vi "Build All TWM Versions.vi"() -> ()   [LabVIEW 2020]
doc: "This VI will automatically build selected versions (different driver sets, etc.)."
uses:
  <vilib>/AppBuilder/AB_API_Simple/Build Specification Version.ctl
  Build Setup.ctl
  1a084e9b-14bd-426b-b511-56d3df6ad0ad.vi
  <vilib>/Utility/error.llb/Error Cluster From Error Code.vi
  <vilib>/AppBuilder/AB_API_Simple/Get Build Specification Version (path).vi
  <vilib>/AppBuilder/AB_API_Simple/Set Build Specification Version (path).vi
  <vilib>/ErrorRing/Error Ring.xnode
  <vilib>/Comparison/Equal/Equal Functor/Equal Functor.lvclass
  <vilib>/AppBuilder/AB_API_Simple/NI_App_Builder_API.lvlib
panel:
  in  "btn exit":bool
  in  "Build Specification Version (editable)":T1
  in  "build regexp filter":string="TWM -" caption="Build Specification regexp Filter (e.g.: \"TWM-\" or \".*\" for no filtering)"
  out "Status":string
  in  "btn all":bool
  in  "builds":i32[](listbox) caption="Available build variants (different configuration sets, select some for build):"
  in  "Target Name":string="My Computer" caption="Target Name (typically \"My Computer\")"
  in  "full build name":string="TWM - full" caption="Build Specification Name (the fully equiped version)"
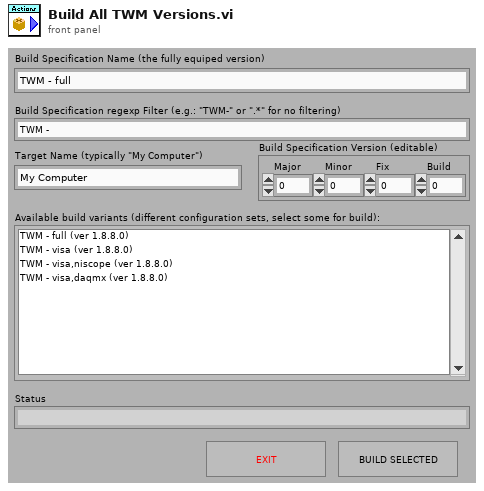
[diagram p1: front panel]
types:
  T1 = typedef "NI_App_Builder_API.lvlib/Build Specification Version.ctl" = cluster{"Major":u16, "Minor":u16, "Fix":u16, "Build":u16}
  T2 = typedef "Build Setup.ctl" = cluster{"project path":path, "build spec name":string, "target name":string}
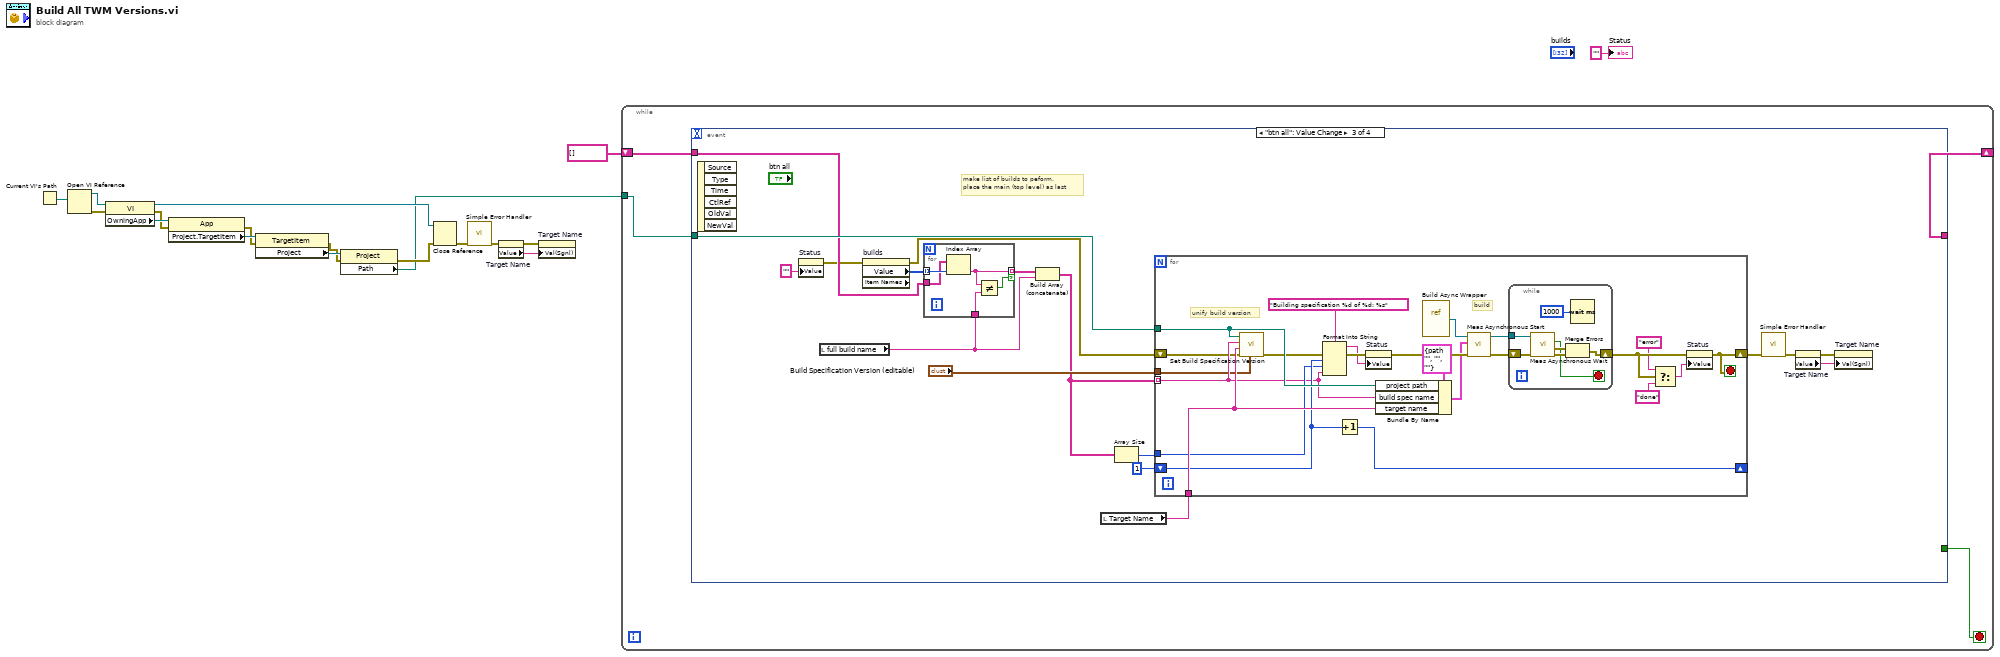
[diagram p0: block diagram]
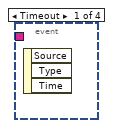
[diagram p2: hidden frame]
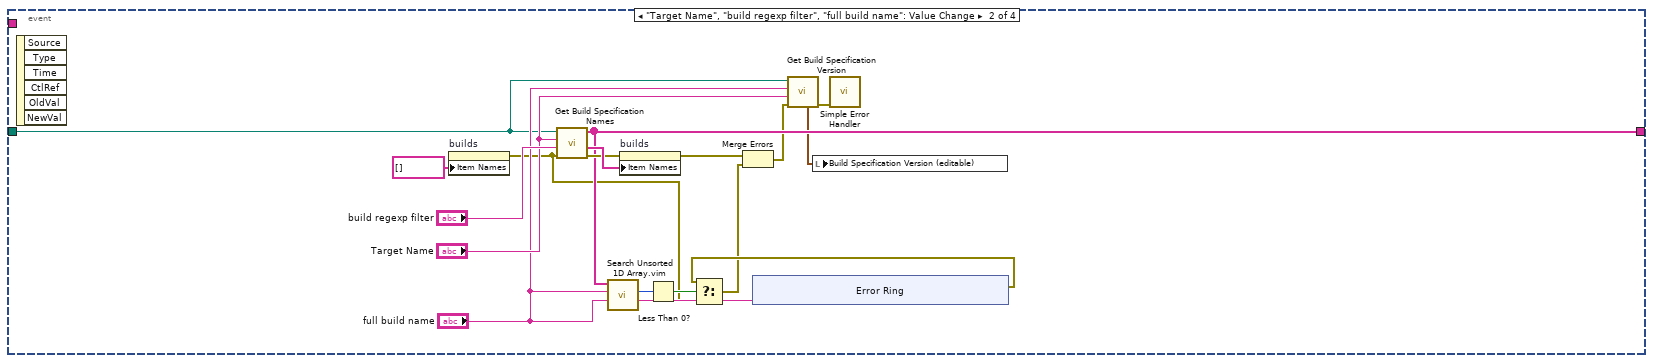
[diagram p3: hidden frame]
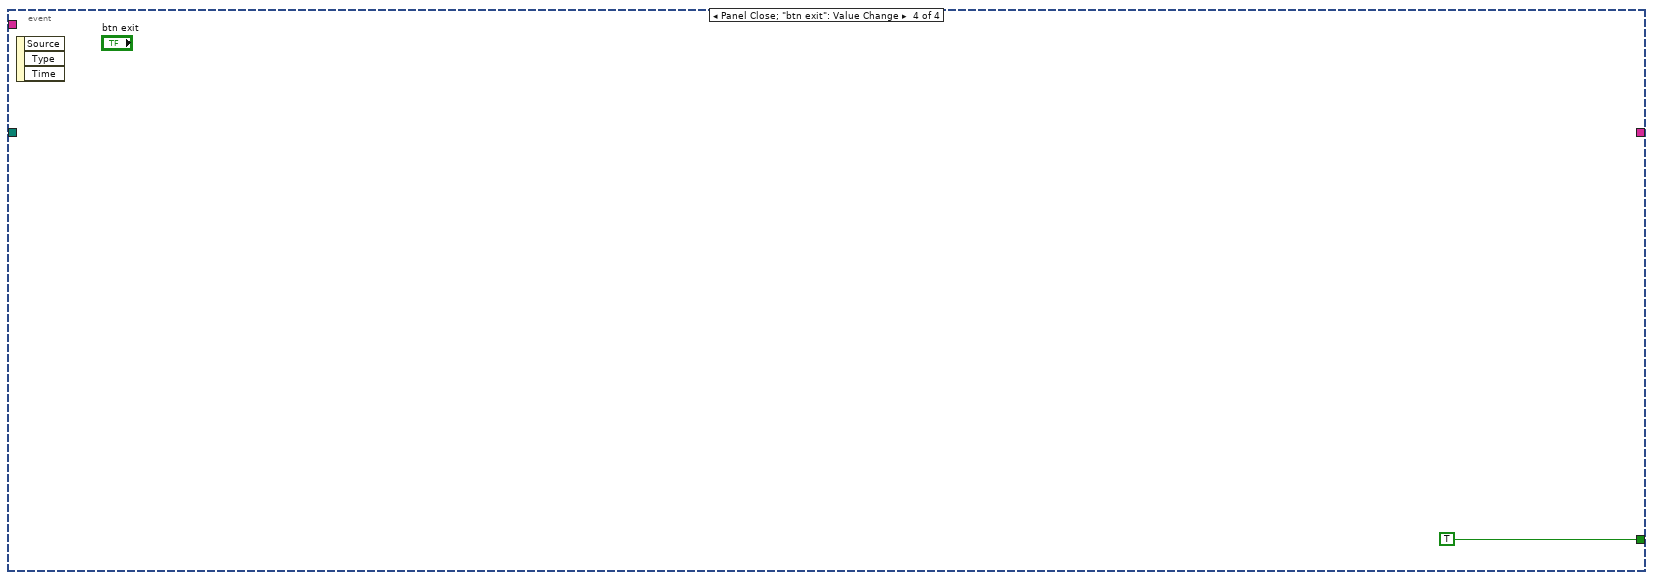
[diagram p4: hidden frame]
diagram:
  n1 = Current VI's Path() -> (path=w17:path)
  n2 = Open VI Reference(vi path=w17) -> (vi reference=w15:refnum<vi>, error out=w16:errorcluster)  [unwired: 5 in]
  n3 = property class="VI"(reference=w15, error in=w16) -> (reference out=w10:refnum<vi>, error out=w13:errorcluster, "OwningApp"=w14:refnum<vi>)
  n4 = property class="App"(reference=w14, error in=w13) -> (error out=w11:errorcluster, "Project.TargetItem"=w12:refnum<vi>)  [unwired: 1 out]
  n5 = property class="TargetItem"(reference=w12, error in=w11) -> (error out=w8:errorcluster, "Project"=w9:refnum<vi>)  [unwired: 1 out]
  n6 = property class="Project"(reference=w9, error in=w8) -> (error out=w7:errorcluster, "Path"=w6:path)  [unwired: 1 out]
  n7 = Close Reference(reference=w10, error in (no error)=w7) -> (error out=w5:errorcluster)
  n8 = call <vilib>:"Simple Error Handler.vi"("error in (no error)"=w5) -> ("error out"=w3:errorcluster)  [unwired: 4 in, 4 out]
  n9 = property on="Target Name" class="Str"(error in=w3) -> (error out=w1:errorcluster, "Value"=w2:string)  [unwired: 1 in, 1 out]
  n10 = property on="Target Name" class="Str"(error in=w1, "Val(Sgnl)"=w2) -> ()  [unwired: 1 in, 2 out]
  n11 = while {
    tunnel: w6 -> [w22]
    shift-right: [w21] -> _
    shift-left: string[] [] ("Build specification names") -> [w20]
    stop <- w19 stop-if-true
    n12 = event shown="[2] \"btn all\": Value Change" {
      selector: _ -> [_ _ _ _]
      dyn-events: _ -> [_ _ _ _]
      timeout: _ -> [_ _ _ _]
      tunnel: [_ w35 _ _] -> w21
      tunnel: w22 -> [_ w26 w54 _]
      tunnel: w20 -> [_ _ w52 _]
      tunnel: [_ _ _ TRUE] -> w19
      event Timeout {
        n13 = event-data() -> ()  [unwired: 1 in, 3 out]
      }
      event "Target Name", "build regexp filter", "full build name": Value Change {
        n14 = event-data() -> ()  [unwired: 1 in, 6 out]
        n15 = property on="builds" class="LstBox (strict)"("Item Names"=string[] []) -> (error out=w27:errorcluster)  [unwired: 2 in, 1 out]
        n16 = call "Get Build Specification Names.vi"("error in (no error)"=w27, "Build specification regexp filter (.*)"="build regexp filter", "Target Name"="Target Name", "Project Path"=w26) -> ("error out"=w38:errorcluster, "Build specification names with version string"=w39:string[], "Build specification names"=w35:string[])  [unwired: 3 in, 2 out]
        n17 = call "Search Unsorted 1D Array.vim"("element"="full build name", "unsorted 1D array"=w35) -> ("index of element"=w32:i32)  [unwired: 9 in]
        n18 = property on="builds" class="LstBox (strict)"(error in=w38, "Item Names"=w39) -> (error out=w29:errorcluster)  [unwired: 1 in, 1 out]
        n19 = Less Than 0?(x=w32) -> (x < 0?=w31:bool)
        n20 = xnode "Error Ring"("parameter 0"="full build name") -> ("error out"=w30:errorcluster)
        n21 = Select(t=w30, s=w31, f=w27) -> (s? t:f=w28:errorcluster)
        n22 = Merge Errors(w29, w28) -> (w25:errorcluster)
        n23 = call-poly <vilib>:"Get Build Specification Version.vi"("error in (no error)"=w25, "Name of target (My Computer)"="Target Name", "Name of build specification"="full build name", "Path to project"=w26) -> ("error out"=w24:errorcluster, "Build Specification Version"=w23:T1)  [unwired: 6 in]
        n24 = local write "Build Specification Version (editable)"(w23) -> ()
        n25 = call <vilib>:"Simple Error Handler.vi"("error in (no error)"=w24) -> ()  [unwired: 4 in, 5 out]
      }
      event "btn all": Value Change {
        # "make list of builds to peform,\nplace the main (top level) as last"
        n26 = event-data() -> ()  [unwired: 1 in, 6 out]
        n27 = property on="Status" class="Str"("Value"="" ("Status")) -> (error out=w48:errorcluster)  [unwired: 2 in, 1 out]
        n28 = local read "full build name"() -> (w62:string)
        n29 = property on="builds" class="LstBox (strict)" props=["Value", "Item Names"](error in=w48) -> (error out=w60:errorcluster, "Value"=w56:i32[])  [unwired: 1 in, 2 out]
        n30 = for {
          tunnel: w56 -> [w98] mode=indexing
          tunnel: w52 -> [w97]
          tunnel: w62 -> [w96]
          tunnel: [w95] -> w58 mode=indexing if=w94
          n31 = Index Array(array=w97, index=w98) -> (element=w95:string)
          n32 = Not Equal?(x=w95, y=w96) -> (x != y?=w94:bool)
        }
        n33 = Build Array (concatenate)(w58, w62) -> (w59:string[])
        n34 = local read "Target Name"() -> (w63:string)
        n35 = Array Size(array=w59) -> (size(s)=w57:i32)
        n36 = for {
          tunnel: w54 -> [w86]
          tunnel: w63 -> [w85]
          tunnel: w59 -> [w71] mode=indexing
          tunnel: w57 -> [w72]
          shift-right: [w84] -> _
          shift-left: 1 -> [w73]
          shift-right: [w68] -> w55
          shift-left: w60 -> [w69]
          tunnel: "Build Specification Version (editable)" -> [w70]
          stop <- w68 stop-if-true
          # "build"
          # "unify build version"
          n37 = call-poly <vilib>:"Set Build Specification Version.vi"("Build Specification Version"=w70, "error in (no error)"=w69, "Name of target (My Computer)"=w85, "Name of build specification"=w71, "Path to project"=w86) -> ("error out"=w82:errorcluster)  [unwired: 6 in]
          n38 = Format Into String(format string="Building specification %d of %d: %s", error in=w82, w73, w72, w71) -> (resulting string=w80:string, error out=w83:errorcluster)  [unwired: 1 in]
          n39 = Increment(x=w73) -> (x+1=w84:i32)
          n40 = property on="Status" class="Str"(error in=w83, "Value"=w80) -> (error out=w79:errorcluster)  [unwired: 1 in, 1 out]
          n41 = Bundle By Name(cluster=T2 {"project path"=path "", "build spec name"="", "target name"=""} ("build setup"), "project path"=w86, "build spec name"=w71, "target name"=w85) -> (w77:T2)
          n42 = vi-ref "Build Async Wrapper.vi"() -> (w76:refnum<vi>)
          n43 = call "Meas Asynchronous Start.vi"("error in"=w79, "parameter in"=w77, "Static VI reference in (empty)"=w76) -> ("error out"=w75:errorcluster, "async VI reference out"=w74:refnum<vi>)  [unwired: 7 in]
          n44 = while {
            tunnel: w74 -> [w92]
            shift-right: [w89] -> w67
            shift-left: w75 -> [w93]
            stop <- w88 stop-if-true
            n45 = call "Meas Asynchronous Wait.vi"("error in"=w93, "VI reference (empty)"=w92) -> ("error out"=w91:errorcluster, "VI's error out"=w90:errorcluster, "VI returned?"=w88:bool)  [unwired: 5 in, 2 out]
            n46 = Merge Errors(w90, w91) -> (w89:errorcluster)
            n47 = Wait (ms)(milliseconds to wait=u32 1000) -> ()  [unwired: 1 out]
          }
          n48 = Select(t="error" ("Status"), s=w67, f="done" ("Status")) -> (s? t:f=w64:string)
          n49 = property on="Status" class="Str"(error in=w67, "Value"=w64) -> (error out=w68:errorcluster)  [unwired: 1 in, 1 out]
        }
        n50 = call <vilib>:"Simple Error Handler.vi"("error in (no error)"=w55) -> ("error out"=w49:errorcluster)  [unwired: 4 in, 4 out]
        n51 = property on="Target Name" class="Str"(error in=w49) -> (error out=w51:errorcluster, "Value"=w50:string)  [unwired: 1 in, 1 out]
        n52 = property on="Target Name" class="Str"(error in=w51, "Val(Sgnl)"=w50) -> ()  [unwired: 1 in, 2 out]
      }
      event Panel Close; "btn exit": Value Change {
        n53 = event-data() -> ()  [unwired: 1 in, 3 out]
      }
    }
  }
  "Status" <- "" ("Status")
